vi "FindFolder to LV Path.vi"(2 "error in (no error)":errorcluster, 3 "CreateFolder (false)":bool, 4 "FindFolderType":T1=enum."kPreferencesFolderType", 5 "FindFolderDomain (UserDomain)":T2=enum."kUserDomain") -> (0 "error out":errorcluster, 1 "LV Path":path)   [LabVIEW 2020]
uses:
  <vilib>/Platform/FileManager.llb/FindFolderDomain.ctl
  <vilib>/Platform/FileManager.llb/FindFolderType.ctl
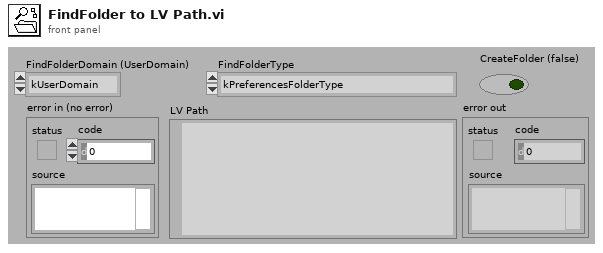
[diagram p1: front panel]
types:
  T1 = typedef "FindFolderType.ctl" = enum16{"kSystemFolderType", "kDesktopFolderType", "kSystemDesktopFolderType", "kTrashFolderType", "kSystemTrashFolderType", "kWhereToEmptyTrashFolderType", "kPrintMonitorDocsFolderType", "kStartupFolderType", "kShutdownFolderType", "kAppleMenuFolderType", "kControlPanelFolderType", "kSystemControlPanelFolderType", "kExtensionFolderType", "kFontsFolderType", "kPreferencesFolderType", "kSystemPreferencesFolderType", "kTemporaryFolderType", "kExtensionDisabledFolderType", "kControlPanelDisabledFolderType", "kSystemExtensionDisabledFolderType", "kStartupItemsDisabledFolderType", "kShutdownItemsDisabledFolderType", "kApplicationsFolderType", "kDocumentsFolderType", "kVolumeRootFolderType", "kChewableItemsFolderType", "kApplicationSupportFolderType", "kTextEncodingsFolderType", "kStationeryFolderType", "kOpenDocFolderType", "kOpenDocShellPlugInsFolderType", "kEditorsFolderType", "kOpenDocEditorsFolderType", "kOpenDocLibrariesFolderType", "kGenEditorsFolderType", "kHelpFolderType", "kInternetPlugInFolderType", "kModemScriptsFolderType", "kPrinterDescriptionFolderType", "kPrinterDriverFolderType", "kScriptingAdditionsFolderType", "kSharedLibrariesFolderType", "kVoicesFolderType", "kControlStripModulesFolderType", "kAssistantsFolderType", "kUtilitiesFolderType", "kAppleExtrasFolderType", "kContextualMenuItemsFolderType", "kMacOSReadMesFolderType", "kALMModulesFolderType", "kALMPreferencesFolderType", "kALMLocationsFolderType", "kColorSyncProfilesFolderType", "kThemesFolderType", "kFavoritesFolderType", "kInternetFolderType", "kAppearanceFolderType", "kSoundSetsFolderType", "kDesktopPicturesFolderType", "kInternetSearchSitesFolderType", "kFindSupportFolderType", "kFindByContentFolderType", "kInstallerLogsFolderType", "kScriptsFolderType", "kFolderActionsFolderType", "kLauncherItemsFolderType", "kRecentApplicationsFolderType", "kRecentDocumentsFolderType", "kRecentServersFolderType", "kSpeakableItemsFolderType", "kKeychainFolderType", "kQuickTimeExtensionsFolderType", "kDisplayExtensionsFolderType", "kMultiprocessingFolderType", "kPrintingPlugInsFolderType", "kDomainTopLevelFolderType", "kDomainLibraryFolderType", "kColorSyncFolderType", "kColorSyncCMMFolderType", "kColorSyncScriptingFolderType", "kPrintersFolderType", "kSpeechFolderType", "kCarbonLibraryFolderType", "kDocumentationFolderType", "kDeveloperDocsFolderType", "kDeveloperHelpFolderType", "kISSDownloadsFolderType", "kUserSpecificTmpFolderType", "kCachedDataFolderType", "kFrameworksFolderType", "kPrivateFrameworksFolderType", "kClassicDesktopFolderType", "kDeveloperFolderType", "kSystemSoundsFolderType", "kComponentsFolderType", "kQuickTimeComponentsFolderType", "kCoreServicesFolderType", "kPictureDocumentsFolderType", "kMovieDocumentsFolderType", "kMusicDocumentsFolderType", "kInternetSitesFolderType", "kPublicFolderType", "kAudioSupportFolderType", "kAudioSoundsFolderType", "kAudioSoundBanksFolderType", "kAudioAlertSoundsFolderType", "kAudioPlugInsFolderType", "kAudioComponentsFolderType", "kKernelExtensionsFolderType", "kDirectoryServicesFolderType", "kDirectoryServicesPlugInsFolderType", "kInstallerReceiptsFolderType", "kFileSystemSupportFolderType", "kAppleShareSupportFolderType", "kAppleShareAuthenticationFolderType", "kMIDIDriversFolderType", "kKeyboardLayoutsFolderType", "kIndexFilesFolderType", "kFindByContentIndexesFolderType", "kManagedItemsFolderType", "kBootTimeStartupItemsFolderType", "kLocalesFolderType", "kFindByContentPluginsFolderType", "kUsersFolderType", "kCurrentUserFolderType", "kCurrentUserRemoteFolderLocation", "kCurrentUserRemoteFolderType", "kSharedUserDataFolderType", "kVolumeSettingsFolderType", "kAppleshareAutomountServerAliasesFolderType", "kPreMacOS91ApplicationsFolderType", "kPreMacOS91InstallerLogsFolderType", "kPreMacOS91AssistantsFolderType", "kPreMacOS91UtilitiesFolderType", "kPreMacOS91AppleExtrasFolderType", "kPreMacOS91MacOSReadMesFolderType", "kPreMacOS91InternetFolderType", "kPreMacOS91AutomountedServersFolderType", "kPreMacOS91StationeryFolderType"}
  T2 = typedef "FindFolderDomain.ctl" = enum16{"kSystemDomain", "kLocalDomain", "kNetworkDomain", "kUserDomain", "kClassicDomain"}
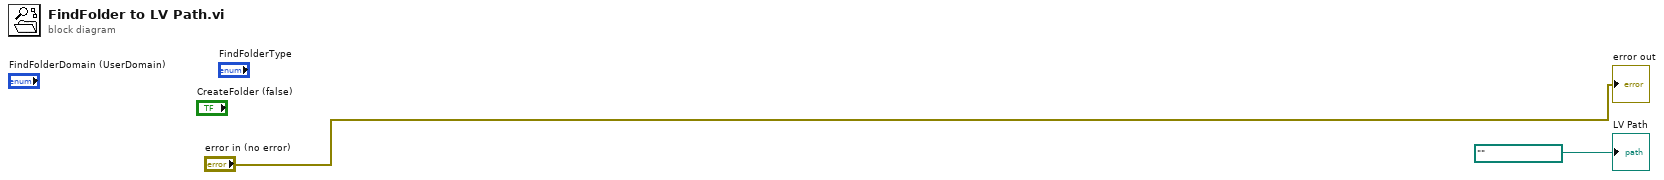
[diagram p0: block diagram]
diagram:
  "error out" <- "error in (no error)"
  "LV Path" <- path "" ("LV Path")
